vi "GrabPlotImage.vi"(11 "WaveformGraph in":refnum<vi>) -> ()   [LabVIEW 2022 SP3]
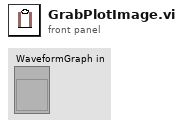
[diagram p1: front panel]
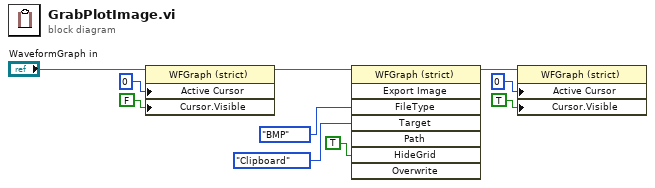
[diagram p0: block diagram]
diagram:
  n1 = property on="Property Node" class="WFGraph (strict)"(reference="WaveformGraph in", "Active Cursor"=u32 0, "Cursor.Visible"=FALSE) -> (reference out=w1:refnum<vi>)  [unwired: 1 in, 1 out]
  n2 = invoke class="WFGraph (strict)" method="Export Image"(reference=w1, "FileType"=enum32{"BMP", "EPS", "EMF", "PICT"}."BMP" ("File Type"), "Target"=enum32{"File", "Clipboard"}."Clipboard", "HideGrid"=TRUE ("Hide Grid")) -> (reference out=w2:refnum<vi>)  [unwired: 4 in, 7 out]
  n3 = property on="Property Node" class="WFGraph (strict)"(reference=w2, "Active Cursor"=u32 0, "Cursor.Visible"=TRUE) -> ()  [unwired: 1 in, 2 out]
